vi "Dialog Tester - Format String.vi"() -> ()   [LabVIEW 2019]
doc: "<b>TEST VI</b> checks for string formatting verification"
uses:
  <vilib>/Utility/config.llb/Read Key (String).vi
  Popup/Popup.lvclass
  <vilib>/Utility/config.llb/NI_LVConfig.lvlib
panel:
  out "read from file":string
  in  "File?":bool
  out "String Test":string
  in  "String Input":string="<b><i>BOLD</i></b>\n<i>italic</i>\n<strong>Strong</strong>\n<del>strike</del>\n<em>emphasis</em>\n<ins>underline</ins>\n<font rgb(0, 0, 255)><b>blue</b></font> other text\n<font rgb(0, 255, 0)><b>green</b></font>\n<font rgb(255, 0, 0)>red</font>"
  # "<[bi]>|\n<strong>|\n<del>|\n<em>|\n<ins>|\n<font rgb(.*?)>"
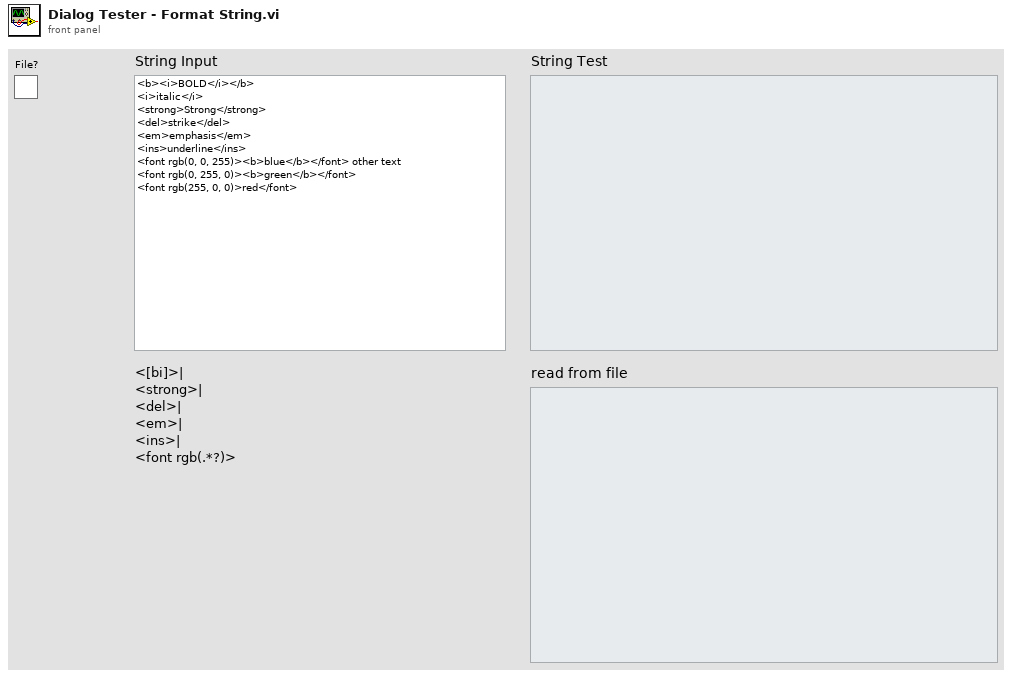
[diagram p1: front panel]
types:
  T1 = typedef "NI_LVConfig.lvlib/Config Data RefNum.ctl" = refnum<k1>
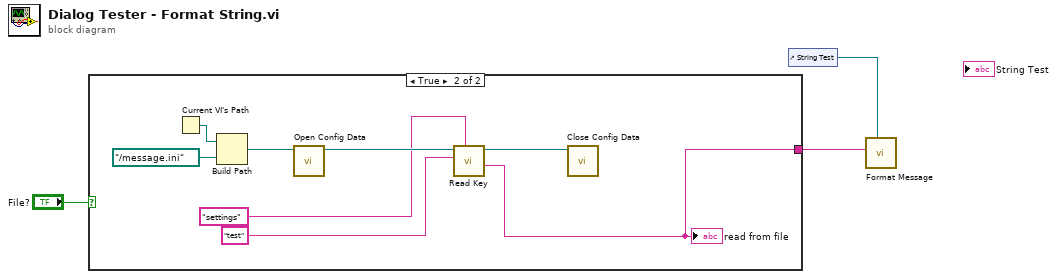
[diagram p0: block diagram]
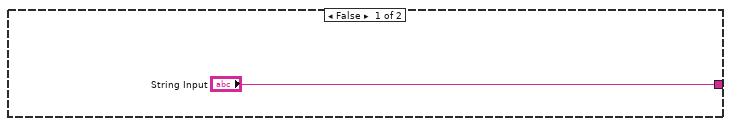
[diagram p2: hidden frame]
diagram:
  n1 = case shown="True" "File?" {
    tunnel: ["String Input" w5] -> w1
    frame False {
    }
    frame True {
      n2 = Current VI's Path() -> (path=w11:path)
      n3 = Build Path(base path=w11, name or relative path=path "../message.ini") -> (appended path=w12:path)
      n4 = call <vilib>:"Open Config Data.vi"("configuration file path"=w12) -> ("refnum"=w9:T1)  [unwired: 8 in, 2 out]
      n5 = call-poly <vilib>:"Read Key.vi"("section"="settings", "key"="test" ("section"), "refnum"=w9) -> ("value"=w5:string, "refnum out"=w8:T1)  [unwired: 5 in, 2 out]
      "read from file" <- w5
      n6 = call <vilib>:"Close Config Data.vi"("refnum"=w8) -> ()  [unwired: 9 in, 2 out]
    }
  }
  n7 = control-ref of="String Test"() -> (w3:refnum<vi>)
  n8 = call "Format Message.vi"("formatted string"=w3, "String Input"=w1) -> ()  [unwired: 8 in, 2 out]
